vi "Read N.vi"(8 "error in (no error)":errorcluster, 11 "Online_TRAC in":refnum<class "Online_TRAC.lvclass">) -> (0 "error out":errorcluster, 2 "N":u64, 3 "Online_TRAC out":refnum<class "Online_TRAC.lvclass">)   [LabVIEW 2021, in "Online_TRAC.lvclass"]
uses:
  Online_TRAC.lvclass
  Online_TRAC.lvclass/Online_TRAC.ctl
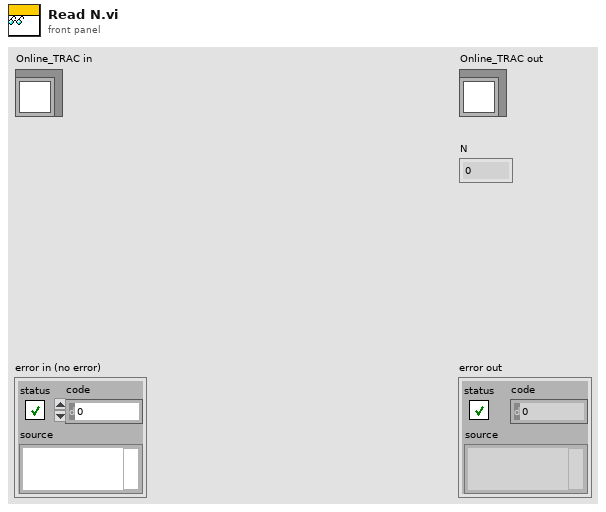
[diagram p1: front panel]
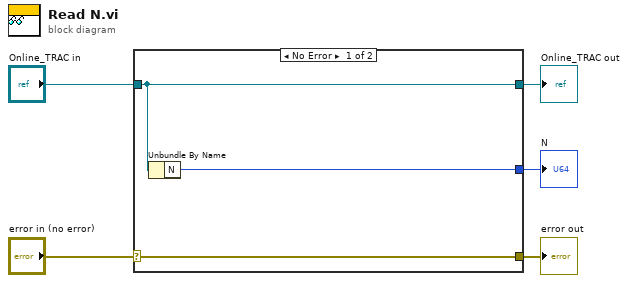
[diagram p0: block diagram]
diagram:
  n1 = case shown="No Error" "error in (no error)" {
    selector: "error in (no error)" -> [w8 w9]
    tunnel: [w8 w9] -> w4
    tunnel: [w7 w10] -> w2
    tunnel: "Online_TRAC in" -> [w7 w10]
    tunnel: [w6 _] -> w1
    frame No Error {
      n2 = Unbundle By Name(w7) -> ("N"=w6:u64)
    }
    frame Error {
    }
  }
  "error out" <- w4
  "Online_TRAC out" <- w2
  "N" <- w1
